vi "Move AxisX DistY.vi"() -> ()   [LabVIEW 2015]
uses:
  <userlib>/Newport ESP301/Newport ESP301.lvlib
panel:
  in  "Axis":i32
  in  "Movement":dbl
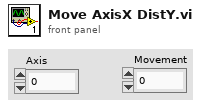
[diagram p1: front panel]
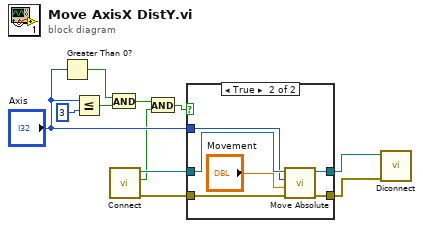
[diagram p0: block diagram]
diagram:
  n1 = Greater Than 0?(x="Axis") -> (x > 0?=w9:bool)
  n2 = Less Or Equal?(x="Axis", y=3) -> (x <= y?=w10:bool)
  n3 = And(x=w9, y=w10) -> (x .and. y?=w8:bool)
  n4 = call "Connect.vi"() -> ("error out"=w4:errorcluster, "Connected"=w3:bool, "VISA resource name out"=w5:refnum<visa-resource-name>)  [unwired: 5 in]
  n5 = And(x=w8, y=w3) -> (x .and. y?=w7:bool)
  n6 = case shown="True" w7 {
    tunnel: w5 -> [w13 w18]
    tunnel: w4 -> [w12 w19]
    tunnel: [w13 w14] -> w2
    tunnel: [w12 w15] -> w1
    tunnel: "Axis" -> [_ w16]
    frame False {
    }
    frame True {
      n7 = call <userlib>:"Move Absolute.vi"("error in (no error)"=w19, "Position (0 units)"="Movement", "Axis (1)"=w16, "VISA resource name"=w18) -> ("error out"=w15:errorcluster, "VISA resource name out"=w14:refnum<visa-resource-name>)  [unwired: 2 in]
    }
  }
  n8 = call "Diconnect.vi"("error in (no error)"=w1, "VISA resource name"=w2) -> ()  [unwired: 6 in]
